vi "gfitsio-read-column-datetime.vi"(6 "row":i32, 7 "column":string, 8 "error in (no error)":errorcluster, 11 "gfits refnum":T1) -> (0 "error out":errorcluster, 2 "data":timestamp, 3 "dup gfits refnum":T1)   [LabVIEW 2011, in "gfitsio.lvlib"]
doc: "Read elements from an ASCII or binary table column."
uses:
  gfitsio.lvlib
  gfitsio-refnum.ctl
  cfitsio-hdutypes.ctl
  gfitsio.dll
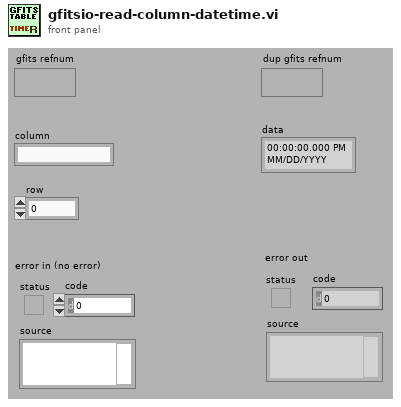
[diagram p1: front panel]
types:
  T1 = typedef "gfitsio.lvlib/gfitsio-refnum.ctl" = refnum<k1>
  T2 = typedef "gfitsio.lvlib/cfitsio-hdutypes.ctl" = i32
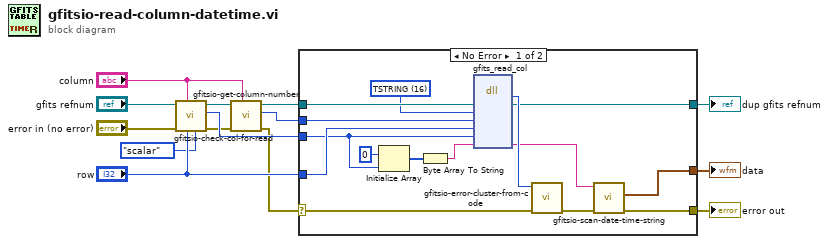
[diagram p0: block diagram]
diagram:
  n1 = call "gfitsio-check-col-for-read.vi"("expected dimensionality"=enum16{"scalar", "array"}."scalar", "row"="row", "column"="column", "error in (no error)"="error in (no error)", "gfits refnum"="gfits refnum") -> ("error out"=w5:errorcluster, "nelements"=w8:i32, "dup gfits refnum"=w7:T1)  [unwired: 4 in]
  n2 = call "gfitsio-get-column-number.vi"("column"="column", "error in (no error)"=w5, "gfits refnum"=w7) -> ("error out"=w4:errorcluster, "colnum"=w3:i32, "dup gfits refnum"=w6:T1)  [unwired: 6 in]
  n3 = case shown="No Error" w4 {
    selector: w4 -> [w29 w31]
    tunnel: [w17 w31] -> w14
    tunnel: w6 -> [w26 w30]
    tunnel: [w27 w30] -> w13
    tunnel: "row" -> [w24 _]
    tunnel: w3 -> [w25 _]
    tunnel: [w15 _] -> w12
    tunnel: w8 -> [w22 _]
    frame No Error {
      w23 = T2 16 items=["TBIT"=1, "TBYTE  (U8)"=11, "TSBYTE  (I8)"=12, "TLOGICAL"=14, "TSTRING"=16, "TUSHORT  (U16)"=20, "TSHORT  (I16)"=21, "TUINT"=31, "TULONG  (U32)"=40, "TLONG  (I32)"=41, "TFLOAT  (SGL)"=42, "TLONGLONG  (I64)"=81, "TDOUBLE"=82, "TCOMPLEX  (CSG)"=83, "TDOUBLECOMPLEX  (CDB)"=163] ("cfitsio datatype")
      n4 = Initialize Array(u8 0, w22) -> (w20:u8[])
      n5 = Byte Array To String(unsigned byte array=w20) -> (string=w19:string)
      n6 = dll-call lib="C:/BonOMM/BonOMM-SAOMM/SubVIs/gfitsio/gfitsio.dll" fn="gfits_read_col"("dup gfits refnum"=w26, "datatype"=w23, "colnum"=w25, "row"=w24, "nelements"=w22, "data"=w19) -> (w28:i32, "dup gfits refnum"=w27:T1, "data"=w16:string)  [unwired: 7 in, 2 out]
      n7 = call "gfitsio-error-cluster-from-code.vi"("error in (no error)"=w29, "error code"=w28) -> ("error out"=w18:errorcluster)  [unwired: 9 in]
      n8 = call "gfitsio-scan-date-time-string.vi"("error in (no error)"=w18, "date/time string"=w16) -> ("error out"=w17:errorcluster, "timestamp"=w15:timestamp)  [unwired: 8 in]
    }
    frame Error {
    }
  }
  "error out" <- w14
  "dup gfits refnum" <- w13
  "data" <- w12
